vi "Get Flow Rate.vi"(8 "error in":errorcluster, 11 "CPC in":refnum<class "CPC.lvclass">) -> (0 "error out":errorcluster, 2 "Q":dbl, 3 "CPC out":refnum<class "CPC.lvclass">)   [LabVIEW 2014, in "CPC.lvclass"]
uses:
  CPC.lvclass
  Controls/CmdStruct.ctl
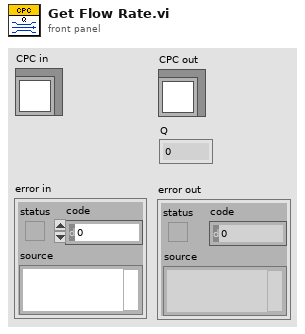
[diagram p1: front panel]
types:
  T1 = typedef "CmdStruct.ctl" = cluster{"Cmd":u8, "x":i64, "y":i64, "Display":string}
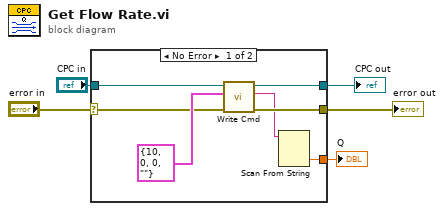
[diagram p0: block diagram]
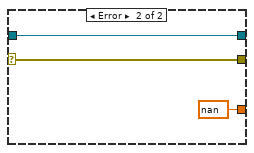
[diagram p2: hidden frame]
diagram:
  n1 = case shown="No Error" "error in" {
    selector: "error in" -> [w10 w15]
    tunnel: [w9 w15] -> w4
    tunnel: [w8 w14] -> w2
    tunnel: "CPC in" -> [w12 w14]
    tunnel: [w6 nan] -> w1
    frame No Error {
      n2 = call-dynamic "Write Cmd.vi"("error in"=w10, "CmdStruct"=T1 {"Cmd"=10, "x"=0, "y"=0, "Display"=""}, "CPC in"=w12) -> ("error out"=w9:errorcluster, "Buffer"=w7:string, "CPC out"=w8:refnum<class "CPC.lvclass">)  [unwired: 6 in]
      n3 = Scan From String(input string=w7) -> (output 1=w6:dbl)  [unwired: 4 in, 3 out]
    }
    frame Error {
    }
  }
  "error out" <- w4
  "CPC out" <- w2
  "Q" <- w1
